vi "Band Integral Separate (SubVI).vi"(8 "Wavelength End":dbl=768.0 min=200.0 max=1100.0 step=1.0, 9 "Wavelength Start":dbl=764.0 min=200.0 max=1100.0 step=1.0, 10 "To Integrate":dbl[](array[numeric]), 11 "Wavelength Array (nm)":dbl[](array[numeric])) -> (2 "Integral":dbl)   [LabVIEW 2018]
uses:
  <vilib>/Analysis/NI_AALPro.lvlib
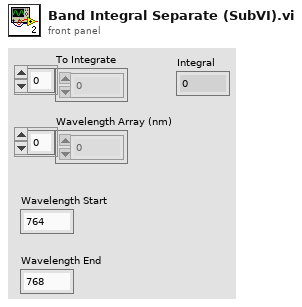
[diagram p1: front panel]
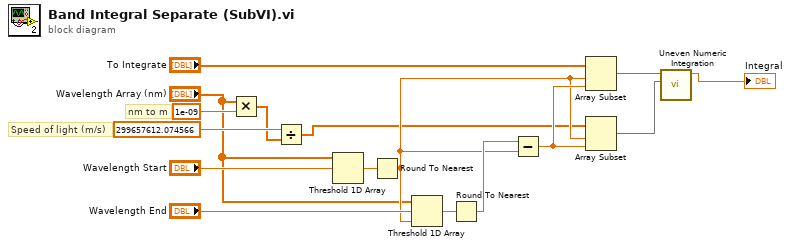
[diagram p0: block diagram]
diagram:
  # "nm to m"
  # "Speed of light (m/s)"
  n1 = Multiply(x="Wavelength Array (nm)", y=1e-09) -> (x*y=w3:dbl[])
  n2 = Divide(x=299657612.074566, y=w3) -> (x/y=w2:dbl[])
  n3 = Threshold 1D Array(2:"Wavelength Start", 3:"Wavelength Array (nm)") -> (0:w14:dbl)  [unwired: 1 in]
  n4 = Round To Nearest(number=w14) -> (nearest integer value=w8:dbl)
  n5 = Threshold 1D Array(1:w8, 2:"Wavelength End", 3:"Wavelength Array (nm)") -> (0:w13:dbl)
  n6 = Round To Nearest(number=w13) -> (nearest integer value=w11:dbl)
  n7 = Subtract(x=w11, y=w8) -> (x-y=w9:dbl)
  n8 = Array Subset(array="To Integrate", index=w8, length=w9) -> (w12:dbl[])
  n9 = Array Subset(array=w2, index=w8, length=w9) -> (w7:dbl[])
  n10 = call <vilib>:"Uneven Numeric Integration.vi"("T"=w7, "X"=w12) -> ("result"=→"Integral":dbl)  [unwired: 8 in, 1 out]
